vi "extract roi 3d.vi"(9 "ROI selected":i16, 10 "ROIs Array In":i32[][](array[numeric]), 11 "Data Form":T1) -> (2 "Table ROI 3D":i32[][][](array[numeric]))   [LabVIEW 2023]
uses:
  control/Data Form.ctl
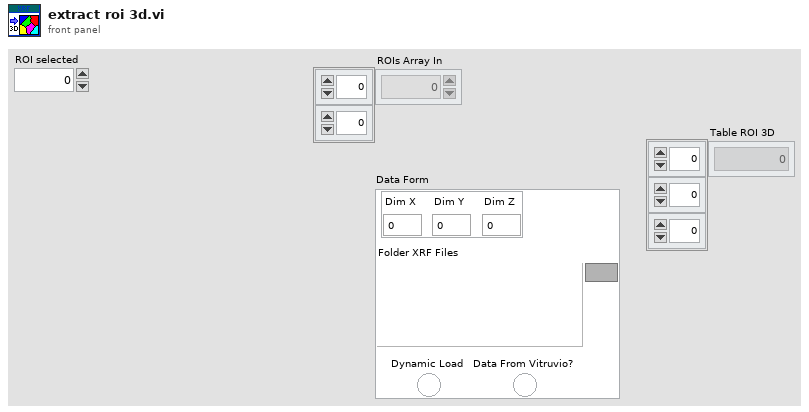
[diagram p1: front panel]
types:
  T1 = typedef "Data Form.ctl" = cluster{"Dimensions":cluster{"Dim X":i32, "Dim Y":i32, "Dim Z":i32}, "Folder XRF Files":path, "Dynamic Load":bool, "Data From Vitruvio?":bool}
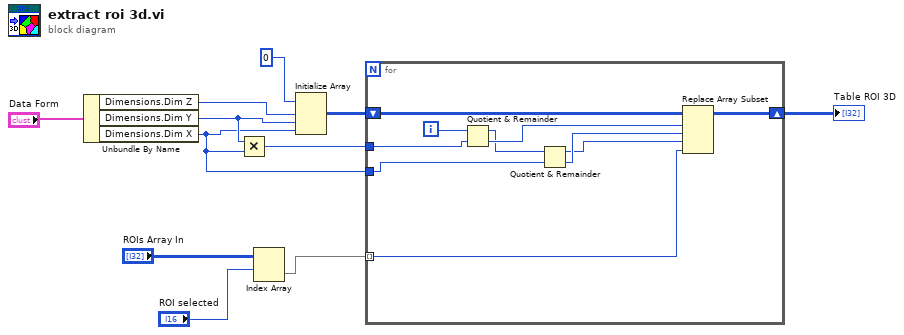
[diagram p0: block diagram]
diagram:
  n1 = Unbundle By Name("Data Form") -> ("Dimensions.Dim Z"=w6:i32, "Dimensions.Dim Y"=w5:i32, "Dimensions.Dim X"=w4:i32)
  n2 = Multiply(x=w5, y=w4) -> (x*y=w7:i32)
  n3 = Index Array(array="ROIs Array In", index (row)="ROI selected") -> (element=w1:i32[])  [unwired: 1 in]
  n4 = Initialize Array(0 ("element"), w6, w5, w4) -> (w9:i32[][][])
  n5 = for {
    tunnel: w1 -> [w18] mode=indexing
    shift-right: [w20] -> w8
    shift-left: w9 -> [w21]
    tunnel: w4 -> [w13]
    tunnel: w7 -> [w12]
    i -> [w19]
    n6 = Quotient & Remainder(x=w19, y=w12) -> (x-y*floor(x/y)=w16:i32, floor(x/y)=w17:i32)
    n7 = Quotient & Remainder(x=w16, y=w13) -> (x-y*floor(x/y)=w14:i32, floor(x/y)=w15:i32)
    n8 = Replace Array Subset(array=w21, new element=w18, index (dim 0)=w17, index (dim 1)=w15, index (dim 2)=w14) -> (w20:i32[][][])
  }
  "Table ROI 3D" <- w8
